vi "题目二.vi"() -> ()   [LabVIEW 2017]
panel:
  in  "Digital Waveform":digitalwaveform(waveform)={"t0"=timestamp(0 s since 1904-01-01), "dt"=1.0, "Y"={"transitions"=[], "data"=[]}} caption="数字波形"
  out "数字波形图":digitalwaveform(graph)
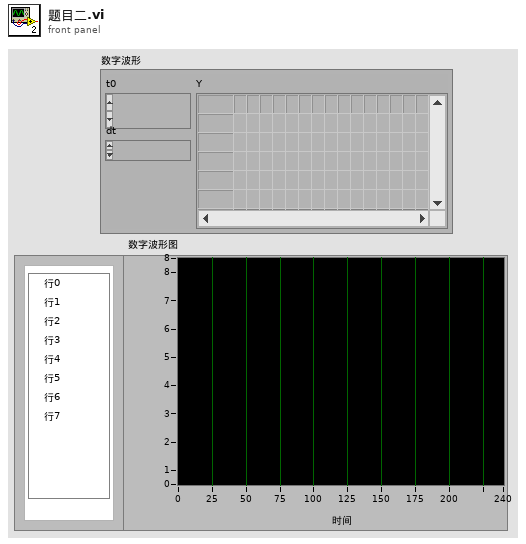
[diagram p1: front panel]
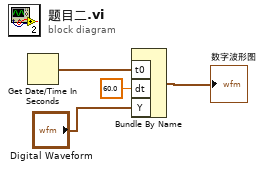
[diagram p0: block diagram]
diagram:
  n1 = Get Date/Time In Seconds() -> (seconds since 1Jan1904=w4:timestamp)
  n2 = Bundle By Name("t0"=w4, "dt"=60.0, "Y"="Digital Waveform") -> (→"数字波形图":digitalwaveform)  [unwired: 1 in]
